vi "z_param.vi"(0 "EOS":T1 items=["Ideal", "CH4_van_der_Waal", "CH4_Redlich_Kwong", "CO2_van_der_Waal", "CO2_Redlich_Kwong", ""]) -> (1 "z_Param_T":dbl[](array[numeric]), 2 "z_Param_P":dbl[](array[numeric]))   [LabVIEW 2016]
uses:
  EOS.ctl
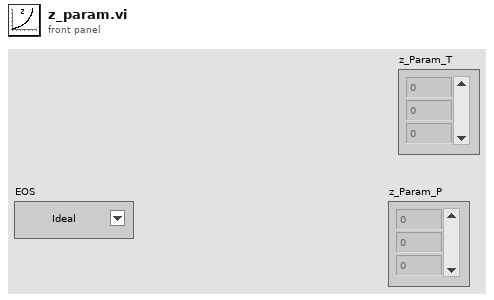
[diagram p1: front panel]
types:
  T1 = typedef "EOS.ctl" = u16
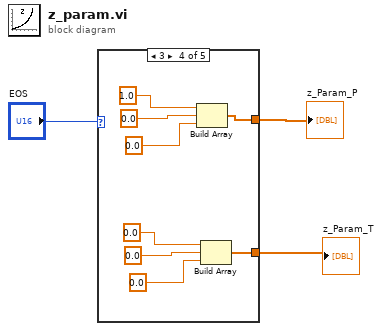
[diagram p0: block diagram]
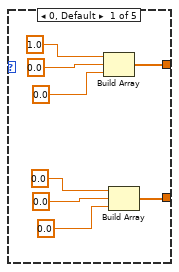
[diagram p2: hidden frame]
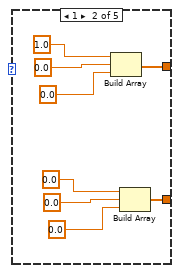
[diagram p3: hidden frame]
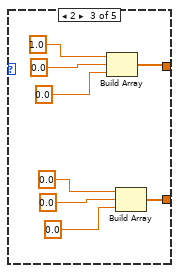
[diagram p4: hidden frame]
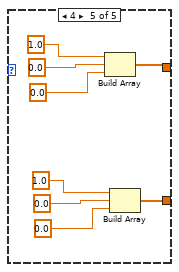
[diagram p5: hidden frame]
diagram:
  n1 = case shown="3" "EOS" {
    tunnel: [w8 w16 w24 w32 w40] -> w2
    tunnel: [w4 w12 w20 w28 w36] -> w1
    frame 0, Default {
      n2 = Build Array(1.0 ("element"), 0.0 ("element"), 0.0 ("element")) -> (w8:dbl[])
      n3 = Build Array(0.0 ("element"), 0.0 ("element"), 0.0 ("element")) -> (w4:dbl[])
    }
    frame 1 {
      n4 = Build Array(1.0 ("element"), 0.0 ("element"), 0.0 ("element")) -> (w16:dbl[])
      n5 = Build Array(0.0 ("element"), 0.0 ("element"), 0.0 ("element")) -> (w12:dbl[])
    }
    frame 2 {
      n6 = Build Array(1.0 ("element"), 0.0 ("element"), 0.0 ("element")) -> (w24:dbl[])
      n7 = Build Array(0.0 ("element"), 0.0 ("element"), 0.0 ("element")) -> (w20:dbl[])
    }
    frame 3 {
      n8 = Build Array(1.0 ("element"), 0.0 ("element"), 0.0 ("element")) -> (w32:dbl[])
      n9 = Build Array(0.0 ("element"), 0.0 ("element"), 0.0 ("element")) -> (w28:dbl[])
    }
    frame 4 {
      n10 = Build Array(1.0 ("element"), 0.0 ("element"), 0.0 ("element")) -> (w40:dbl[])
      n11 = Build Array(1.0 ("element"), 0.0 ("element"), 0.0 ("element")) -> (w36:dbl[])
    }
  }
  "z_Param_P" <- w2
  "z_Param_T" <- w1
